vi "counter_handling.vi"(8 "scan specification":T1={"x amplitude"=0, "x resolution (pixels)"=0, "x offset fly-forward (iterations)"=0, "x offset fly-back (iterations)"=0, "y resolution (nr. of lines)"=0, "y step size"=0, "iterations per pixel"=0, "number of frames"=0, "y offset (pixels)"=0, "number of y-brake lines  (before y-fly-back)"=0, "number y-brake lines (after y-fly-back)"=0, "number of y-fly-back steps"=8, "lines per z step"=0, "number of z/intensity tuples"=0, "number of repetitions (volumes or planes)"=0}, 10 "counter cluster in":T2, 11 "resonant trigger":bool) -> (2 "counter cluster out":T2)   [LabVIEW 2010]
uses:
  counter_cluster.ctl
  scan_specification_cluster.ctl
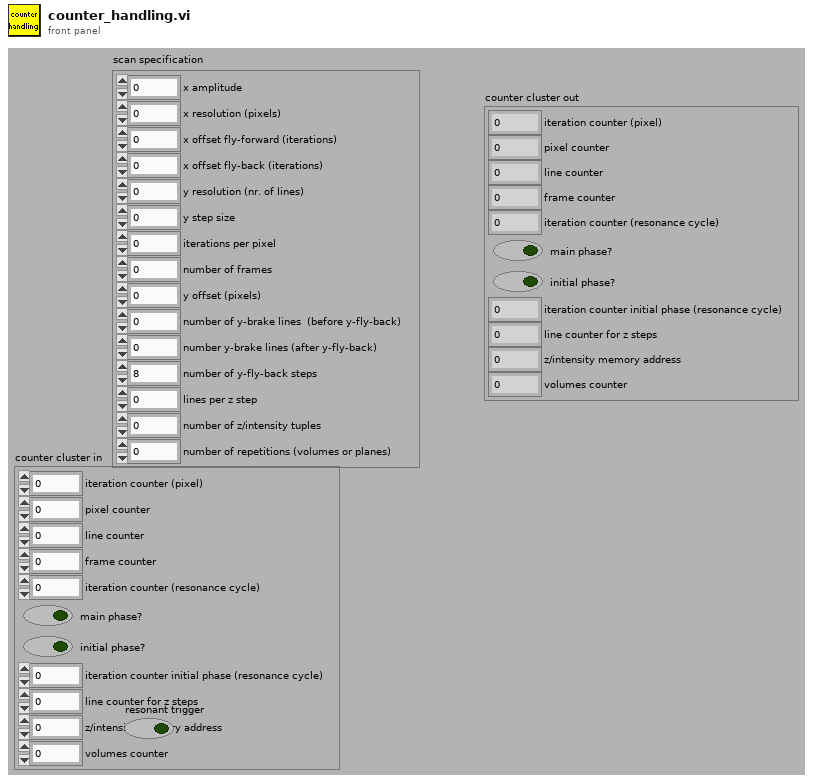
[diagram p1: front panel]
types:
  T1 = typedef "scan_specification_cluster.ctl" = cluster{"x amplitude":u16, "x resolution (pixels)":u16, "x offset fly-forward (iterations)":u16, "x offset fly-back (iterations)":u16, "y resolution (nr. of lines)":u16, "y step size":u16, "iterations per pixel":u16, "number of frames":i32, "y offset (pixels)":u16, "number of y-brake lines  (before y-fly-back)":u16, "number y-brake lines (after y-fly-back)":u16, "number of y-fly-back steps":u16, "lines per z step":u16, "number of z/intensity tuples":u16, "number of repetitions (volumes or planes)":i32}
  T2 = typedef "counter_cluster.ctl" = cluster{"iteration counter (pixel)":u16, "pixel counter":u16, "line counter":u16, "frame counter":u16, "iteration counter (resonance cycle)":u16, "main phase?":bool, "initial phase?":bool, "iteration counter initial phase (resonance cycle)":u16, "line counter for z steps":u16, "z/intensity memory address":u32, "volumes counter":u16}
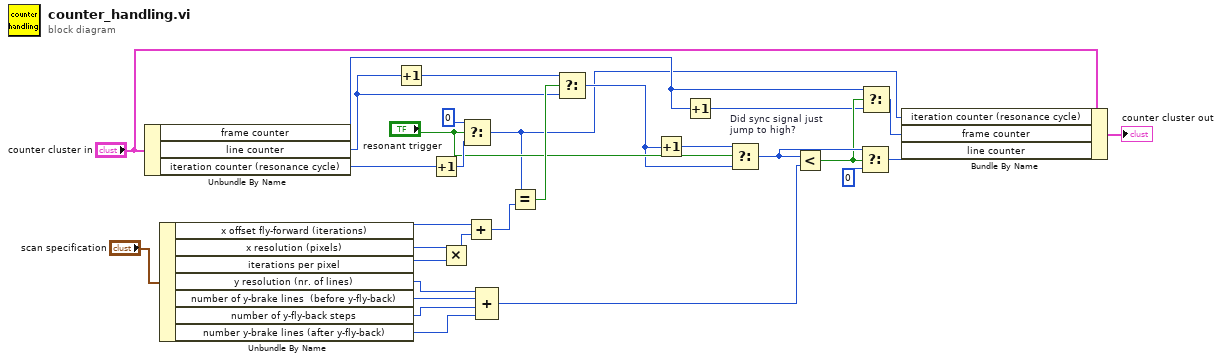
[diagram p0: block diagram]
diagram:
  n1 = Unbundle By Name("counter cluster in") -> ("frame counter"=w17:u16, "line counter"=w14:u16, "iteration counter (resonance cycle)"=w21:u16)
  n2 = Unbundle By Name("scan specification") -> ("x offset fly-forward (iterations)"=w8:u16, "x resolution (pixels)"=w10:u16, "iterations per pixel"=w9:u16, "y resolution (nr. of lines)"=w5:u16, "number of y-brake lines  (before y-fly-back)"=w4:u16, "number of y-fly-back steps"=w3:u16, "number y-brake lines (after y-fly-back)"=w2:u16)
  n3 = Increment(x=w14) -> (x+1=w18:u16)
  n4 = Increment(x=w21) -> (x+1=w20:u16)
  n5 = Multiply(x=w10, y=w9) -> (x*y=w7:u16)
  n6 = Select(t=u16 0 ("f"), s="resonant trigger", f=w20) -> (s? t:f=w12:u16)
  n7 = Add(x=w8, y=w7) -> (x+y=w6:u16)
  n8 = Compound Arithmetic op=ADD(w5, w4, w3, w2) -> (w1:u16)
  n9 = Equal?(x=w12, y=w6) -> (x = y?=w19:bool)
  n10 = Select(t=w18, s=w19, f=w14) -> (s? t:f=w13:u16)
  n11 = Increment(x=w13) -> (x+1=w30:u16)
  n12 = Increment(x=w17) -> (x+1=w23:u16)
  n13 = Select "Did sync signal just\njump to high?"(t=w30, s="resonant trigger", f=w13) -> (s? t:f=w28:u16)
  n14 = Less?(x=w28, y=w1) -> (x < y?=w25:bool)
  n15 = Select(t=w28, s=w25, f=u16 0) -> (s? t:f=w27:u16)
  n16 = Select(t=w17, s=w25, f=w23) -> (s? t:f=w24:u16)
  n17 = Bundle By Name(cluster="counter cluster in", "iteration counter (resonance cycle)"=w12, "frame counter"=w24, "line counter"=w27) -> (→"counter cluster out":T2)
